vi "BGA244_Main.vi"(7 "stop_external":refnum<vi>, 8 "cluster_ref_BGA244":T1) -> ()   [LabVIEW 2019]
uses:
  cluster_ref_BGA244.ctl
panel:
  in  "meas_interval":i32=1000 caption="Measurement interval (ms)"
  out "mode":string
  in  "He/Air Mode Button":bool
  out "Purity Meter":dbl(knob) caption="Purity (%)" scale=0.0..100.0 scale format="%#.2f"
  in  "He Mode Button":bool
  in  "O2/N2 Mode Button":bool
  out "gas 2":string
  out "gas 1":string
  out "Purity Chart":waveform(dbl)[](graph)
  out "Status":bool
  in  "VISA":refnum<visa-resource-name>="COM24"
  out "Last measured":timestamp format="%<%Y-%m-%d %H:%M:%S>T"
  in  "Stop":bool
  # "Gas Analyzer Panel"
  # "1333-74-0: H2\n7440-59-7: He\n7727-37-9: N2\n7782-44-7: O2\n7740-37-1: Ar\n132259-10-0: Air"
  # "BGA244"
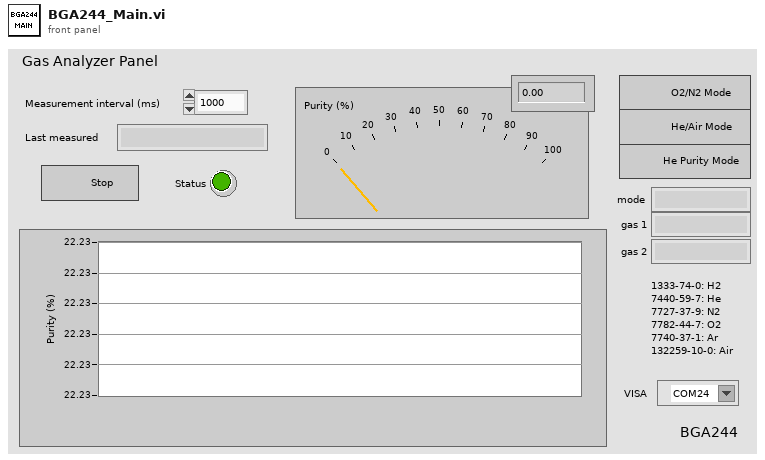
[diagram p1: front panel]
types:
  T1 = typedef "cluster_ref_BGA244.ctl" = cluster{"Status":refnum<vi>, "purity":refnum<vi>}
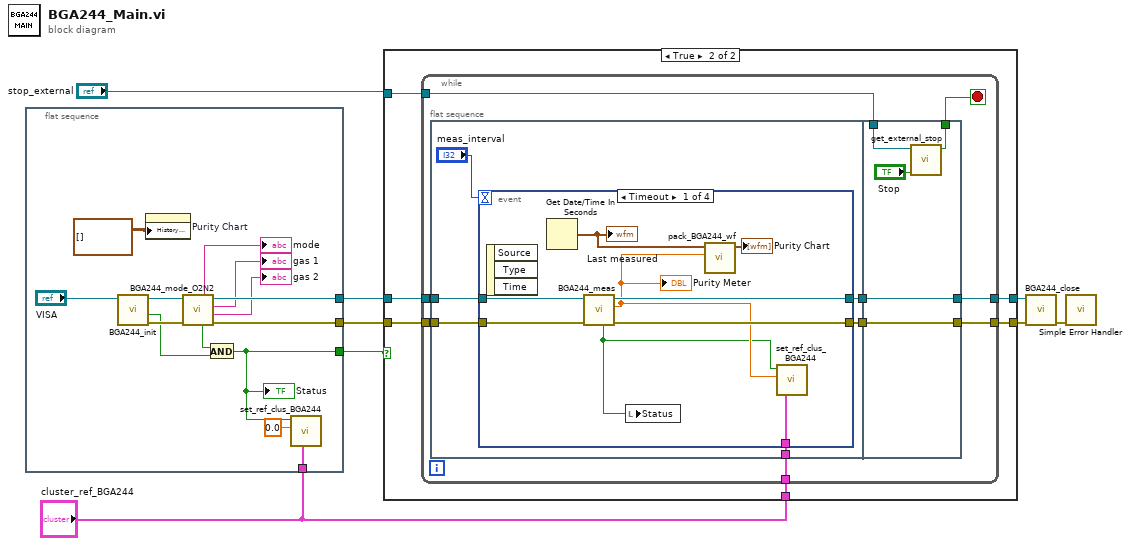
[diagram p0: block diagram]
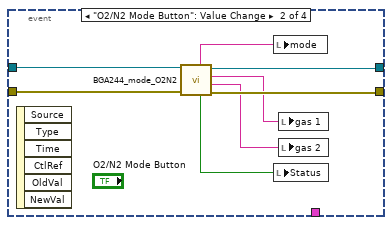
[diagram p3: hidden frame]
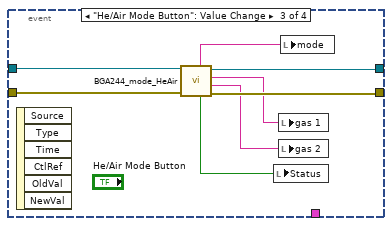
[diagram p4: hidden frame]
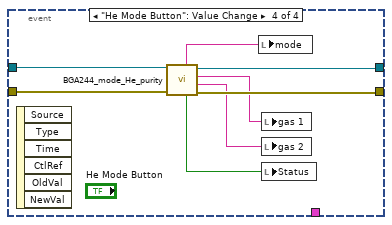
[diagram p5: hidden frame]
diagram:
  n1 = flat-sequence {
    tunnel: [w17] -> w6
    tunnel: [w19] -> w7
    tunnel: "cluster_ref_BGA244" -> [w12]
    tunnel: [w9] -> w1
    frame #0 {
      n2 = call "BGA244_init.vi"("VISA in"="VISA") -> ("error out"=w18:errorcluster, "status"=w14:bool, "VISA out"=w20:refnum<visa-resource-name>)  [unwired: 8 in]
      n3 = property on="Purity Chart" class="WFChart (strict)"("History Data"=waveform(dbl)[][] []) -> ()  [unwired: 2 in, 2 out]
      n4 = call "BGA244_mode_O2N2.vi"("error in"=w18, "VISA in"=w20) -> ("error out"=w17:errorcluster, "gas 2"=→"gas 2":string, "gas 1"=→"gas 1":string, "VISA out"=w19:refnum<visa-resource-name>, "status"=w13:bool, "mode"=→"mode":string)  [unwired: 4 in]
      n5 = And(x=w13, y=w14) -> (x .and. y?=w9:bool)
      "Status" <- w9
      n6 = call "set_ref_clus_BGA244.vi"("cluster_ref_BGA244"=w12, "purity"=0.0, "status"=w9) -> ()  [unwired: 9 in]
    }
  }
  n7 = case shown="True" w1 {
    tunnel: "stop_external" -> [_ w30]
    tunnel: w7 -> [w24 w29]
    tunnel: w6 -> [w23 w28]
    tunnel: [w23 w27] -> w5
    tunnel: [w24 w26] -> w4
    tunnel: "cluster_ref_BGA244" -> [_ w25]
    frame False {
    }
    frame True {
      n8 = while {
        tunnel: w25 -> [w39]
        tunnel: w30 -> [w32]
        tunnel: w29 -> [w38]
        tunnel: w28 -> [w37]
        tunnel: [w36] -> w27
        tunnel: [w35] -> w26
        stop <- w31 stop-if-true
        n9 = flat-sequence {
          tunnel: w39 -> [w45]
          tunnel: w38 -> [w44]
          tunnel: w37 -> [w43]
          tunnel: [w42] -> w34
          tunnel: [w41] -> w33
          tunnel: [w82] -> w35
          tunnel: [w83] -> w36
          tunnel: w34 -> [w83]
          tunnel: w33 -> [w82]
          tunnel: w32 -> [w81]
          tunnel: [w80] -> w31
          frame #0 {
            n10 = event shown="[0] Timeout" {
              selector: _ -> [_ _ _ _]
              dyn-events: _ -> [_ _ _ _]
              timeout: "meas_interval" -> [_ _ _ _]
              tunnel: w45 -> [w54 _ _ _]
              tunnel: w43 -> [w53 w61 w69 w77]
              tunnel: w44 -> [w52 w62 w70 w78]
              tunnel: [w50 w60 w68 w76] -> w41
              tunnel: [w49 w59 w67 w75] -> w42
              event Timeout {
                n11 = event-data() -> ()  [unwired: 1 in, 3 out]
                n12 = Get Date/Time In Seconds() -> (seconds since 1Jan1904=w48:timestamp)
                "Last measured" <- w48
                n13 = call "BGA244_meas.vi"("error in"=w53, "VISA in"=w52) -> ("error out"=w49:errorcluster, "ratio1"=w47:dbl, "VISA out"=w50:refnum<visa-resource-name>, "status"=w46:bool)  [unwired: 5 in, 1 out]
                "Purity Meter" <- w47
                n14 = local write "Status"(w46) -> ()
                n15 = call "pack_BGA244_wf.vi"("purity"=w47, "time"=w48) -> ("waveform_array"=→"Purity Chart":waveform(dbl)[])  [unwired: 9 in]
                n16 = call "set_ref_clus_BGA244.vi"("cluster_ref_BGA244"=w54, "purity"=w47, "status"=w46) -> ()  [unwired: 9 in]
              }
              event "O2/N2 Mode Button": Value Change {
                n17 = event-data() -> ()  [unwired: 1 in, 6 out]
                n18 = call "BGA244_mode_O2N2.vi"("error in"=w61, "VISA in"=w62) -> ("error out"=w59:errorcluster, "gas 2"=w57:string, "gas 1"=w58:string, "VISA out"=w60:refnum<visa-resource-name>, "status"=w56:bool, "mode"=w55:string)  [unwired: 4 in]
                n19 = local write "mode"(w55) -> ()
                n20 = local write "Status"(w56) -> ()
                n21 = local write "gas 1"(w58) -> ()
                n22 = local write "gas 2"(w57) -> ()
              }
              event "He/Air Mode Button": Value Change {
                n23 = event-data() -> ()  [unwired: 1 in, 6 out]
                n24 = call "BGA244_mode_HeAir.vi"("error in"=w69, "VISA in"=w70) -> ("error out"=w67:errorcluster, "gas 2"=w65:string, "gas 1"=w66:string, "VISA out"=w68:refnum<visa-resource-name>, "status"=w64:bool, "mode"=w63:string)  [unwired: 4 in]
                n25 = local write "Status"(w64) -> ()
                n26 = local write "gas 1"(w66) -> ()
                n27 = local write "gas 2"(w65) -> ()
                n28 = local write "mode"(w63) -> ()
              }
              event "He Mode Button": Value Change {
                n29 = event-data() -> ()  [unwired: 1 in, 6 out]
                n30 = call "BGA244_mode_He_purity.vi"("error in"=w77, "VISA in"=w78) -> ("error out"=w75:errorcluster, "gas 2"=w73:string, "gas 1"=w74:string, "VISA out"=w76:refnum<visa-resource-name>, "status"=w72:bool, "mode"=w71:string)  [unwired: 4 in]
                n31 = local write "mode"(w71) -> ()
                n32 = local write "gas 1"(w74) -> ()
                n33 = local write "gas 2"(w73) -> ()
                n34 = local write "Status"(w72) -> ()
              }
            }
          }
          frame #1 {
            n35 = call "get_external_stop.vi"("stop_internal"="Stop", "ref_stop_external"=w81) -> ("stop_output"=w80:bool)  [unwired: 9 in]
          }
        }
      }
    }
  }
  n36 = call "BGA244_close.vi"("error in"=w5, "VISA in"=w4) -> ("error out"=w3:errorcluster)  [unwired: 9 in]
  n37 = call <vilib>:"Simple Error Handler.vi"("error in (no error)"=w3) -> ()  [unwired: 4 in, 5 out]
